vi "createDataNode.vi"(6 "optional":variant, 8 "error in (no error)":errorcluster, 10 "Data Class":string, 11 "xceRootNode in":refnum<class "xceRootNode.lvclass">) -> (0 "error out":errorcluster, 2 "newNode*":refnum<data-value>, 3 "xceRootNode out":refnum<class "xceRootNode.lvclass">)   [LabVIEW 2013, in "xceRootNode.lvclass"]
uses:
  xceRootNode.lvclass
  xceNode/xceNode.lvclass
  xceDataNode/xceDataNode.lvclass
  xceRootNode.lvclass/xceRootNode.ctl
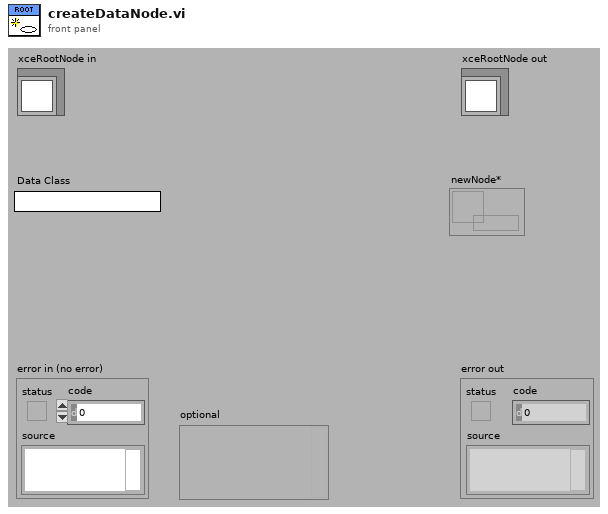
[diagram p1: front panel]
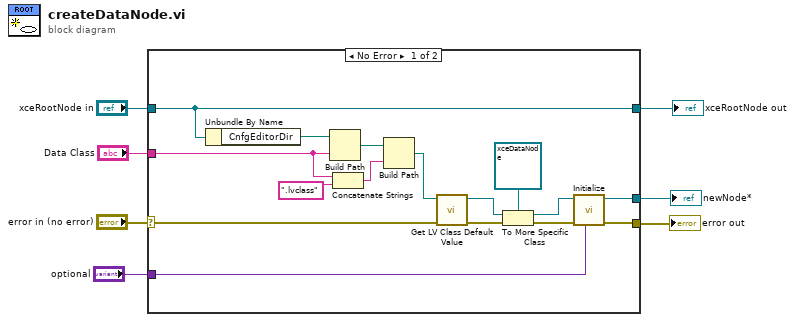
[diagram p0: block diagram]
diagram:
  n1 = case shown="No Error" "error in (no error)" {
    selector: "error in (no error)" -> [w16 w25]
    tunnel: [w9 w25] -> w6
    tunnel: [w23 w24] -> w4
    tunnel: "xceRootNode in" -> [w23 w24]
    tunnel: "Data Class" -> [w21 _]
    tunnel: "optional" -> [w10 _]
    tunnel: [w8 _] -> w1
    frame No Error {
      n2 = Unbundle By Name(w23) -> ("CnfgEditorDir"=w22:path)
      n3 = Build Path(base path=w22, name or relative path=w21) -> (appended path=w19:path)
      n4 = Concatenate Strings(w21, ".lvclass" ("string")) -> (w18:string)
      n5 = Build Path(base path=w19, name or relative path=w18) -> (appended path=w17:path)
      n6 = call <vilib>:"Get LV Class Default Value.vi"("error in (no error)"=w16, "class path"=w17) -> ("error out"=w12:errorcluster, "object"=w15:refnum<class>)  [unwired: 8 in]
      n7 = To More Specific Class(target class=refnum<class "xceDataNode.lvclass"> refnum ("xceDataNode.lvclass"), reference=w15, error in=w12) -> (specific class reference=w13:refnum<class "xceDataNode.lvclass">, error out=w11:errorcluster)
      n8 = call-dynamic "Initialize.vi"("optional"=w10, "error in"=w11, "xceDataNode in"=w13) -> ("error out"=w9:errorcluster, "Node*"=w8:refnum<data-value>)  [unwired: 7 in]
    }
    frame Error {
    }
  }
  "error out" <- w6
  "xceRootNode out" <- w4
  "newNode*" <- w1
